vi "Write for model CNF tcp_ip.vi"(9 "data in":string, 10 "remote port or service name":u16=5000, 11 "address":string="192.168.1.60") -> (0 "error IO":errorcluster, 3 "connection ID":refnum<k5>)   [LabVIEW 2015]
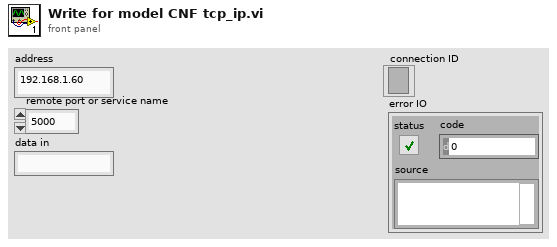
[diagram p1: front panel]
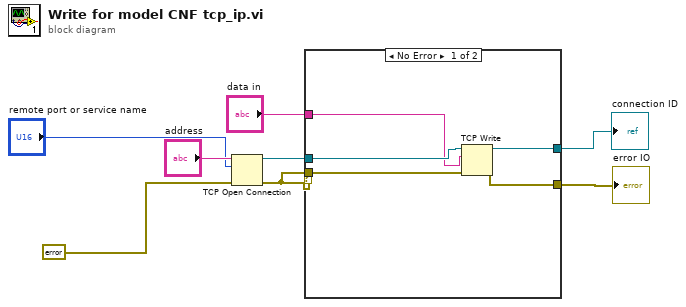
[diagram p0: block diagram]
diagram:
  n1 = TCP Open Connection(address="address", remote port or service name="remote port or service name", error in (no error)=errorcluster {"status"=FALSE, "code"=0, "source"=""}) -> (connection ID=w5:refnum<k5>, error out=w4:errorcluster)  [unwired: 2 in]
  n2 = case shown="No Error" w4 {
    selector: w4 -> [_ w14]
    tunnel: w5 -> [w11 w15]
    tunnel: w4 -> [w10 _]
    tunnel: [w13 w15] -> w2
    tunnel: [w12 w14] -> w1
    tunnel: "data in" -> [w9 _]
    frame No Error {
      n3 = TCP Write(connection ID=w11, data in=w9, error in (no error)=w10) -> (connection ID out=w13:refnum<k5>, error out=w12:errorcluster)  [unwired: 1 in, 1 out]
    }
    frame Error {
    }
  }
  "connection ID" <- w2
  "error IO" <- w1
